vi "温度电阻读取.vi"(8 "error in (no error)":errorcluster, 9 "温度通道":string, 10 "电阻通道":string, 11 "VISA resource name":refnum<visa-resource-name>) -> (0 "error out":errorcluster, 3 "VISA resource name out":refnum<visa-resource-name>)   [LabVIEW 2021]
uses:
  <instrlib>/Keithley DMM6500 DAQ6500 Series/Public/Configure/Configure Temperature (Thermocouple).vi
  <instrlib>/Keithley DMM6500 DAQ6500 Series/Keithley DMM6500 DAQ6500 Series.lvlib
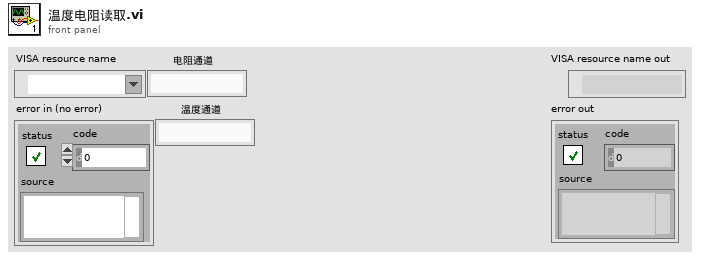
[diagram p1: front panel]
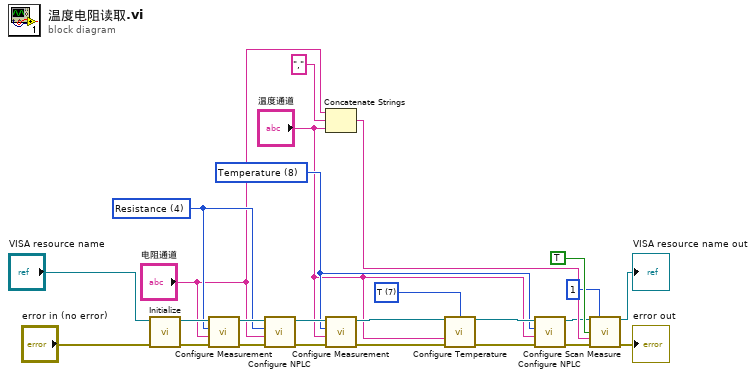
[diagram p0: block diagram]
diagram:
  w15 = 7 items=["B", "E", "J", "K", "N", "R", "S", "T"] ("Thermocouple Type (3: K)")
  w11 = 8 items=["Voltage DC", "Voltage AC", "Current DC", "Current AC", "Resistance", "4-wire Resistance", "Diode", "Capacitance", "Temperature", "Continuity", "Frequency", "Period", "Voltage Ratio", "Voltage", "Current"] ("Function (0: Voltage DC)")
  w19 = 4 items=["Voltage DC", "Voltage AC", "Current DC", "Current AC", "Resistance", "4-wire Resistance", "Diode", "Capacitance", "Temperature", "Continuity", "Frequency", "Period", "Voltage Ratio", "Voltage", "Current"] ("Function (0: Voltage DC)")
  n1 = call <instrlib>:"Initialize.vi"("error in (no error)"="error in (no error)", "VISA resource name"="VISA resource name") -> ("error out"=w22:errorcluster, "VISA resource name out"=w25:refnum<visa-resource-name>)  [unwired: 8 in]
  n2 = call <instrlib>:"Configure Measurement.vi"("error in (no error)"=w22, "Channel List(\"\")"="电阻通道", "Function (0: Voltage DC)"=w19, "VISA resource name"=w25) -> ("error out"=w21:errorcluster, "VISA resource name out"=w20:refnum<visa-resource-name>)  [unwired: 6 in]
  n3 = call <instrlib>:"Configure NPLC.vi"("error in (no error)"=w21, "Channel List(\"\")"="电阻通道", "Function (0: Voltage DC)"=w19, "VISA resource name"=w20) -> ("error out"=w17:errorcluster, "VISA resource name out"=w18:refnum<visa-resource-name>)  [unwired: 6 in]
  n4 = Concatenate Strings("电阻通道", "," ("字符串"), "温度通道") -> (w7:string)
  n5 = call <instrlib>:"Configure Measurement.vi"("error in (no error)"=w17, "Channel List(\"\")"="温度通道", "Function (0: Voltage DC)"=w11, "VISA resource name"=w18) -> ("error out"=w16:errorcluster, "VISA resource name out"=w13:refnum<visa-resource-name>)  [unwired: 6 in]
  n6 = call-poly <instrlib>:"Configure Temperature.vi"("VISA resource name"=w13, "Thermocouple Type (3: K)"=w15, "Channel List(\"\")"="温度通道", "error in (no error)"=w16) -> ("VISA resource name out"=w12:refnum<visa-resource-name>, "error out"=w14:errorcluster)  [unwired: 10 in]
  n7 = call <instrlib>:"Configure NPLC.vi"("error in (no error)"=w14, "Channel List(\"\")"="温度通道", "Function (0: Voltage DC)"=w11, "VISA resource name"=w12) -> ("error out"=w3:errorcluster, "VISA resource name out"=w5:refnum<visa-resource-name>)  [unwired: 6 in]
  n8 = call <instrlib>:"Configure Scan Measure.vi"("VISA resource name"=w5, "Scan Count (0)"=u32 1, "Enable Scan Reset (T: Enable)"=TRUE, "Channel List(\"\")"=w7, "error in (no error)"=w3) -> ("VISA resource name out"=→"VISA resource name out":refnum<visa-resource-name>, "error out"=→"error out":errorcluster)  [unwired: 9 in]
